vi "User Console.vi"(8 "error in":errorcluster) -> (0 "error out":errorcluster)   [LabVIEW 2020]
doc: "User Console thread VI"
uses:
  Controls/Events_User.ctl
  Database/Controls/Account Database.ctl
  Controls/Data_Initialize.ctl
  SubVIs/User Event - Stop/User Event - Stop.lvlib
  <vilib>/Utility/error.llb/Error Cluster From Error Code.vi
  <vilib>/ErrorRing/Error Ring.xnode
  SubVIs/Message Queue/Message Queue.lvlib
  SubVIs/Message Queue/Enqueue Message (Single).vi
  FGV/Controls/FGV_State.ctl
  Controls/User Console references.ctl
  Controls/User console Local Data.ctl
  Controls/Keypad.ctl
  Controls/Transactions.ctl
  Controls/User Console.ctl
panel:
  in  "User Console":T1
  # "[Covers: UI2]"
  # "[Covers: UI1]"
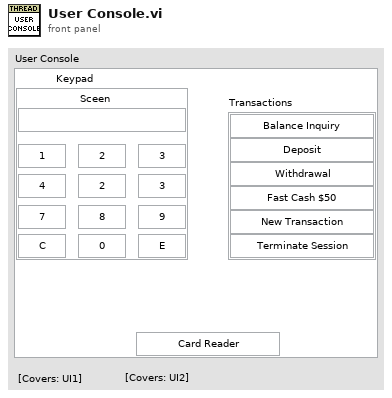
[diagram p1: front panel]
types:
  T1 = typedef "User Console.ctl" = cluster{"Keypad":T2, "Transactions":T3, "Card Reader":bool}
  T2 = typedef "Keypad.ctl" = cluster{"Sceen":string, "1":bool, "2":bool, "3":bool, "4":bool, "5":bool, "6":bool, "7":bool, "8":bool, "9":bool, "C":bool, "0":bool, "E":bool}
  T3 = typedef "Transactions.ctl" = cluster{"Balance Inquiry":bool, "Deposit":bool, "Withdrawal":bool, "Fast Cash $50":bool, "New Transaction":bool, "Terminate Session":bool}
  T4 = enum32{"Invalid", "Standard", "Closed", "Hidden", "Minimized", "Maximized"}
  T5 = typedef "FGV_State.ctl" = enum16{"1 - OpenDatabase", "2 - Initialize Events", "3 - Initialize QMH", "4 - Close QMH", "5 - Close Events", "Read FGV", "Save Database", "Def"}
  T6 = typedef "FGV_Data.ctl" = cluster{"QMH":T7, "User Events":T8, "Database":T9[]}
  T7 = typedef "Message Queue.lvlib/All Message Queues.ctl" = cluster{"User Console":refnum<queue>, "Display Console":refnum<queue>, "Sensor Interface":refnum<queue>, "Process":refnum<queue>}
  T8 = typedef "Events_User.ctl" = cluster{"Stop User Console":refnum<user-event>, "Error User Console":refnum<user-event>, "Stop Sensor Interface ":refnum<user-event>, "Error Sensor Interface":refnum<user-event>}
  T9 = typedef "Account Database.ctl" = cluster{"Account Number":i32, "First Name":string, "Last Name":string, "Balance":dbl}
  T10 = typedef "User console Local Data.ctl" = cluster{"Initiliaze":T11, "User Console Ref":T12, "Configuration Database":T9}
  T11 = typedef "Data_Initialize.ctl" = cluster{"Database":T9[], "User Events":T8}
  T12 = typedef "User Console references.ctl" = cluster{"0":refnum<vi>, "1":refnum<vi>, "2":refnum<vi>, "3":refnum<vi>, "4":refnum<vi>, "5":refnum<vi>, "6":refnum<vi>, "7":refnum<vi>, "8":refnum<vi>, "9":refnum<vi>, "Deposit":refnum<vi>, "Fast Cash $50":refnum<vi>, "Balance Inquiry":refnum<vi>, "Sceen":refnum<vi>, "Card Reader":refnum<vi>, "Withdrawal":refnum<vi>, "New Transaction":refnum<vi>, "Terminate Session":refnum<vi>, "E":refnum<vi>, "C":refnum<vi>}
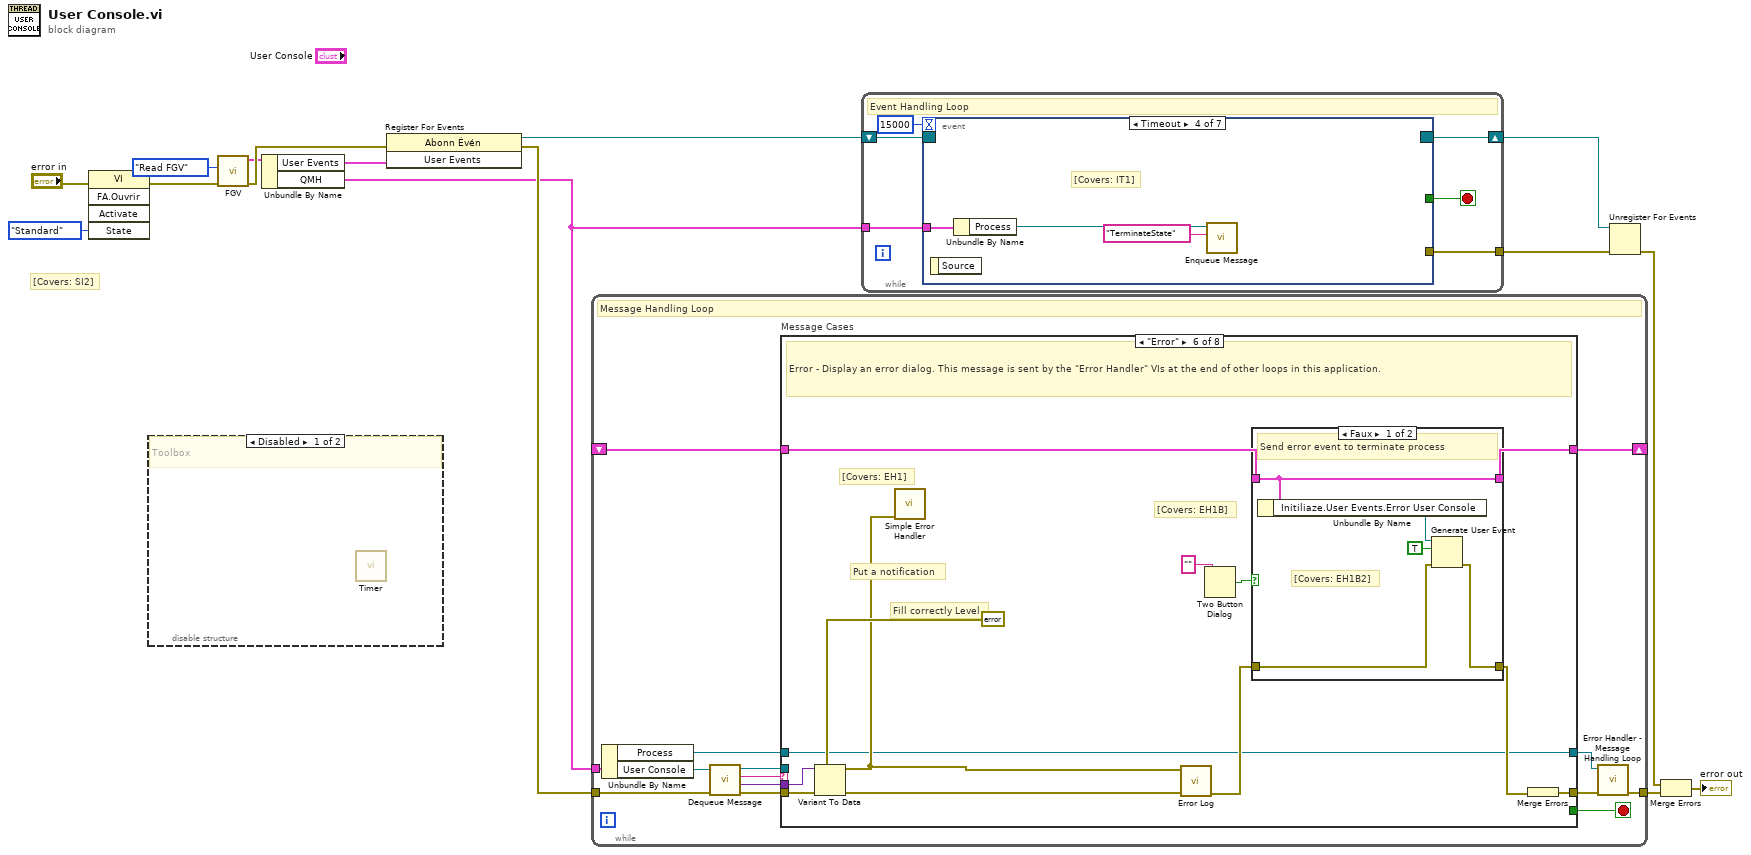
[diagram p0: block diagram]
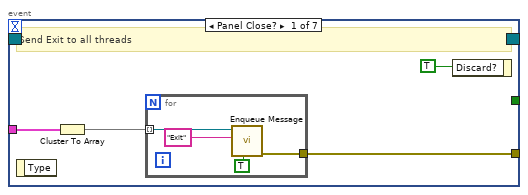
[diagram p3: hidden frame]
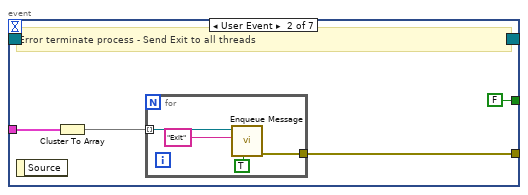
[diagram p4: hidden frame]
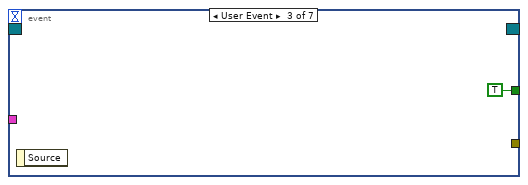
[diagram p5: hidden frame]
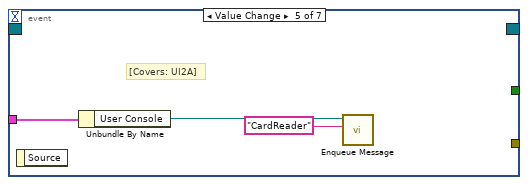
[diagram p6: hidden frame]
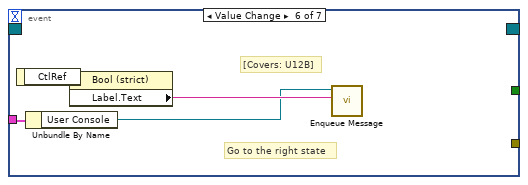
[diagram p7: hidden frame]
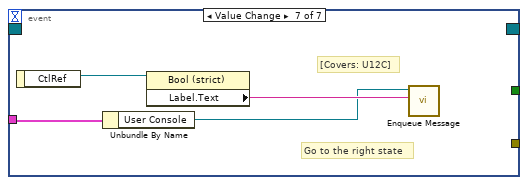
[diagram p8: hidden frame]
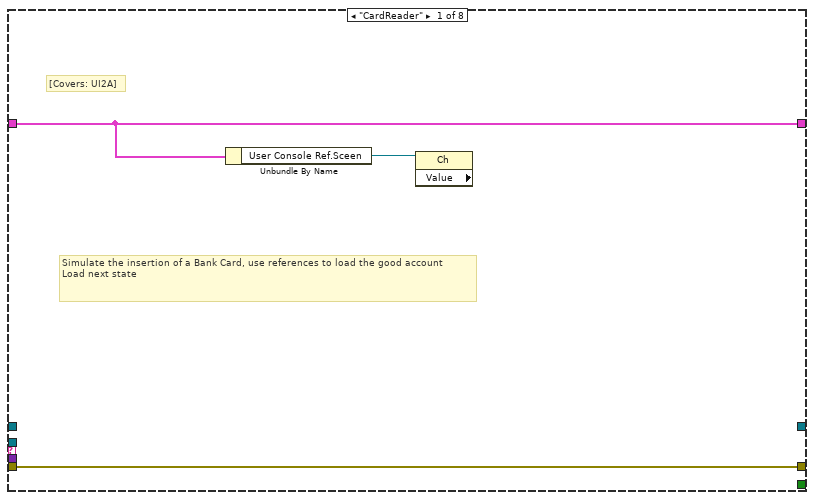
[diagram p9: hidden frame]
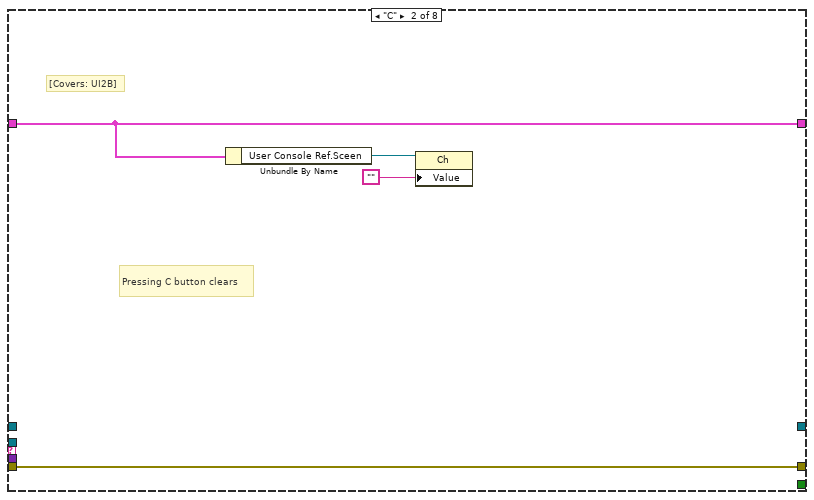
[diagram p10: hidden frame]
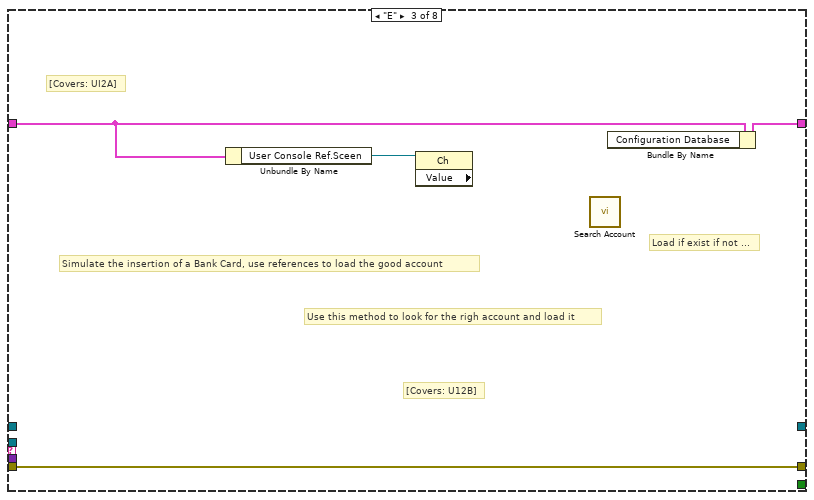
[diagram p11: hidden frame]
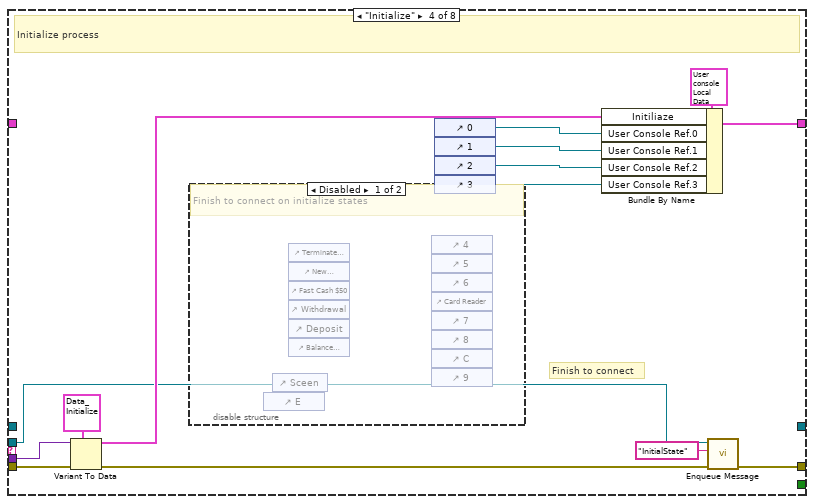
[diagram p12: hidden frame]
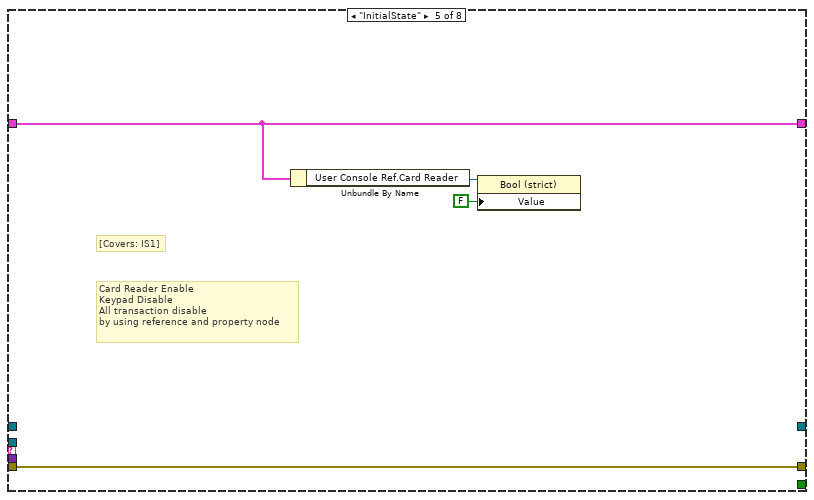
[diagram p14: hidden frame]
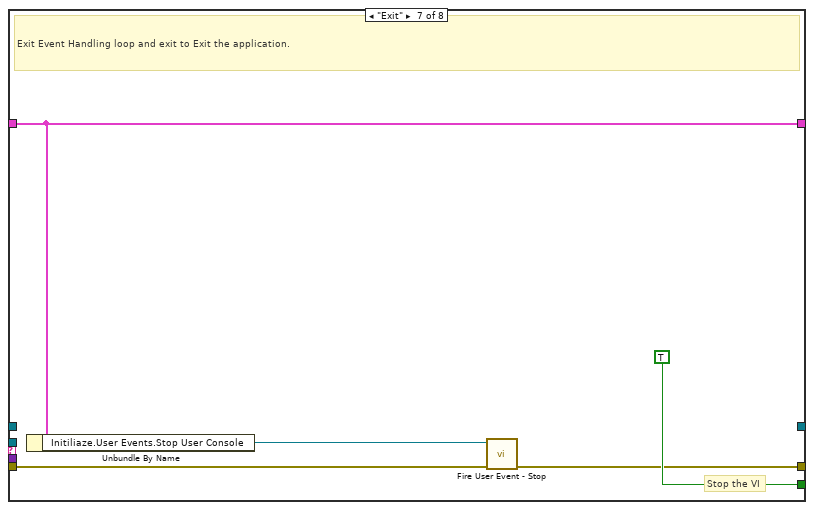
[diagram p16: hidden frame]
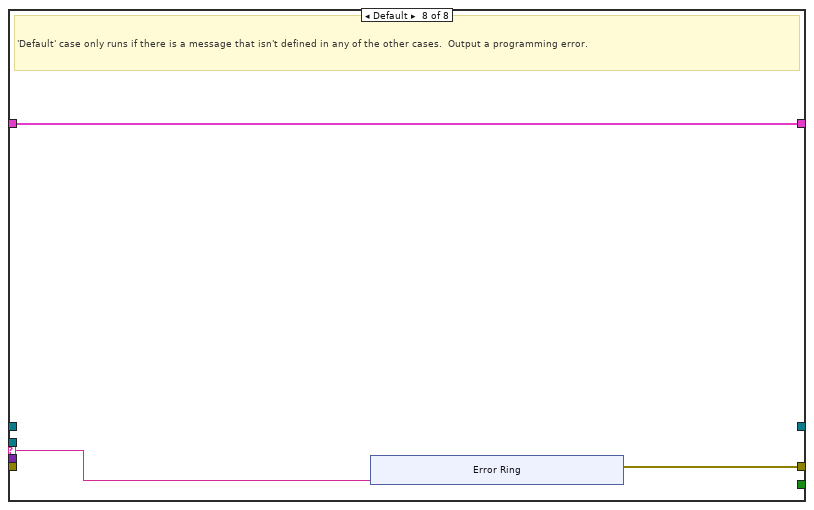
[diagram p17: hidden frame]
diagram:
  # "[Covers: SI2]"
  n1 = invoke class="VI" method="FA.Ouvrir"(error in="error in", "State"=T4."Standard") -> (error out=w2:errorcluster)  [unwired: 3 in, 4 out]
  n2 = disable-structure shown="Disabled" {
    frame Disabled {
      # "Toolbox"
      n3 = call "Timer.vi"() -> ()  [unwired: 9 in, 3 out]
    }
    frame Enabled {
    }
  }
  n4 = call "FGV.vi"("error in (no error)"=w2, "FGV_State"=FGV_State."Read FGV") -> ("error out"=w12:errorcluster, "FGV"=w10:T6)  [unwired: 8 in]
  n5 = Unbundle By Name(w10) -> ("User Events"=w11:T8, "QMH"=w14:T7)
  n6 = register-events(error in=w12, w11) -> (reference out=w8:refnum<event-registration>, error out=w15:errorcluster)  [unwired: 1 in]
  n7 = while {
    tunnel: w14 -> [w19]
    shift-right: [w28] -> _
    shift-left: _ -> [w29]
    tunnel: w15 -> [w26]
    tunnel: [w21] -> w4
    stop <- w27 stop-if-true
    # "Message Handling Loop"
    n8 = Unbundle By Name(w19) -> ("Process"=w17:refnum<queue>, "User Console"=w18:refnum<queue>)
    n9 = call "Dequeue Message.vi"("error in (no error)"=w26, "Message Queue"=w18) -> ("error out"=w25:errorcluster, "Message Data"=w23:variant, "Message"=w24:string, "dup Message Queue"=w22:refnum<queue>)  [unwired: 6 in]
    n10 = case "Message Cases" shown="\"Error\"" w24 {
      selector: w24 -> [_ _ _ _ _ _ _ w84]
      tunnel: w22 -> [_ _ _ w42 _ _ _ _]
      tunnel: w25 -> [w32 w36 w40 w53 w58 w71 w80 _]
      tunnel: [w32 w36 w40 w41 w58 w68 w79 w85] -> w20
      tunnel: w29 -> [w30 w34 w39 _ w57 w62 w82 w86]
      tunnel: [w30 w34 w37 w54 w57 w61 w82 w86] -> w28
      tunnel: [_ _ _ _ _ _ TRUE _] -> w27
      tunnel: w23 -> [_ _ _ w50 _ w70 _ _]
      tunnel: w17 -> [_ _ _ _ _ w59 _ _]
      tunnel: [_ _ _ _ _ w59 _ _] -> w16
      frame "CardReader" {
        # "Simulate the insertion of a Bank Card, use references to load the good account\nLoad next state"
        # "[Covers: UI2A]"
        n11 = Unbundle By Name(w30) -> ("User Console Ref.Sceen"=w31:refnum<vi>)
        n12 = property class="Ch" props=["Value"](reference=w31) -> ()  [unwired: 1 in, 3 out]
      }
      frame "C" {
        # "Pressing C button clears"
        # "[Covers: UI2B]"
        n13 = Unbundle By Name(w34) -> ("User Console Ref.Sceen"=w35:refnum<vi>)
        n14 = property class="Ch"(reference=w35, "Value"="") -> ()  [unwired: 1 in, 2 out]
      }
      frame "E" {
        # "[Covers: U12B]"
        # "Load if exist if not ..."
        # "Use this method to look for the righ account and load it"
        # "Simulate the insertion of a Bank Card, use references to load the good account"
        # "[Covers: UI2A]"
        n15 = Unbundle By Name(w39) -> ("User Console Ref.Sceen"=w38:refnum<vi>)
        n16 = property class="Ch" props=["Value"](reference=w38) -> ()  [unwired: 1 in, 3 out]
        n17 = call "Search Account.vi"() -> ()  [unwired: 9 in, 3 out]
        n18 = Bundle By Name(cluster=w39) -> (w37:T10)  [unwired: 1 in]
      }
      frame "Initialize" {
        # "Finish to connect"
        # "Initialize process"
        n19 = Variant To Data(error in=w53, type=T11 {"Database"=[], "User Events"={"Stop User Console"=refnum, "Error User Console"=refnum, "Stop Sensor Interface "=refnum, "Error Sensor Interface"=refnum}} ("Initiliaze"), Variant=w50) -> (data=w51:T11, error out=w43:errorcluster)
        n20 = disable-structure shown="Disabled" {
          frame Disabled {
            # "Finish to connect on initialize states"
            n21 = control-ref of="E"() -> ()  [unwired: 1 out]
            n22 = control-ref of="Sceen"() -> ()  [unwired: 1 out]
            n23 = control-ref of="Terminate Session"() -> ()  [unwired: 1 out]
            n24 = control-ref of="New Transaction"() -> ()  [unwired: 1 out]
            n25 = control-ref of="Fast Cash $50"() -> ()  [unwired: 1 out]
            n26 = control-ref of="Withdrawal"() -> ()  [unwired: 1 out]
            n27 = control-ref of="Deposit"() -> ()  [unwired: 1 out]
            n28 = control-ref of="Balance Inquiry"() -> ()  [unwired: 1 out]
            n29 = control-ref of="4"() -> ()  [unwired: 1 out]
            n30 = control-ref of="5"() -> ()  [unwired: 1 out]
            n31 = control-ref of="6"() -> ()  [unwired: 1 out]
            n32 = control-ref of="Card Reader"() -> ()  [unwired: 1 out]
            n33 = control-ref of="7"() -> ()  [unwired: 1 out]
            n34 = control-ref of="8"() -> ()  [unwired: 1 out]
            n35 = control-ref of="C"() -> ()  [unwired: 1 out]
            n36 = control-ref of="9"() -> ()  [unwired: 1 out]
          }
          frame Enabled {
          }
        }
        n37 = control-ref of="0"() -> (w48:refnum<vi>)
        n38 = control-ref of="1"() -> (w47:refnum<vi>)
        n39 = control-ref of="2"() -> (w46:refnum<vi>)
        n40 = control-ref of="3"() -> (w45:refnum<vi>)
        n41 = Bundle By Name(cluster=T10 {"Initiliaze"={"Database"=[], "User Events"={"Stop User Console"=refnum, "Error User Console"=refnum, "Stop Sensor Interface "=refnum, "Error Sensor Interface"=refnum}}, "User Console Ref"={"0"=refnum, "1"=refnum, "2"=refnum, "3"=refnum, "4"=refnum, "5"=refnum, "6"=refnum, "7"=refnum, "8"=refnum, "9"=refnum, "Deposit"=refnum, "Fast Cash $50"=refnum, "Balance Inquiry"=refnum, "Sceen"=refnum, "Card Reader"=refnum, "Withdrawal"=refnum, "New Transaction"=refnum, "Terminate Session"=refnum, "E"=refnum, "C"=refnum}, "Configuration Database"={"Account Number"=0, "First Name"="", "Last Name"="", "Balance"=0.0}} ("Local Data"), "Initiliaze"=w51, "User Console Ref.0"=w48, "User Console Ref.1"=w47, "User Console Ref.2"=w46, "User Console Ref.3"=w45) -> (w54:T10)
        n42 = call-poly "Enqueue Message.vi"("error in (no error)"=w43, "Message"="InitialState", "Message Queue"=w42) -> ("error out"=w41:errorcluster)  [unwired: 7 in, 1 out]
      }
      frame "InitialState" {
        # "Card Reader Enable\nKeypad Disable\nAll transaction disable\nby using reference and property node"
        # "[Covers: IS1]"
        n43 = Unbundle By Name(w57) -> ("User Console Ref.Card Reader"=w56:refnum<vi>)
        n44 = property class="Bool (strict)"(reference=w56, "Value"=FALSE) -> ()  [unwired: 1 in, 2 out]
      }
      frame "Error" {
        # "Put a notification"
        # "[Covers: EH1B]"
        # "[Covers: EH1]"
        # "Fill correctly Level"
        # "Error - Display an error dialog. This message is sent by the \"Error Handler\" VIs at the end of other loops in this application."
        n45 = Variant To Data(error in=w71, type=errorcluster {"status"=FALSE, "code"=0, "source"=""} ("error constant"), Variant=w70) -> (data=w66:errorcluster, error out=w67:errorcluster)
        n46 = call <vilib>:"Simple Error Handler.vi"("error in (no error)"=w66) -> ()  [unwired: 4 in, 5 out]
        n47 = call "Error Log.vi"("error in"=w67, "error happened"=w66) -> ("error out"=w65:errorcluster)  [unwired: 9 in]
        n48 = Two Button Dialog(message="") -> (T button?=w64:bool)  [unwired: 2 in]
        n49 = case shown="Faux" w64 {
          tunnel: w65 -> [w74 w78]
          tunnel: [w73 w78] -> w63
          tunnel: w62 -> [w76 w77]
          tunnel: [w76 w77] -> w61
          frame False {
            # "[Covers: EH1B2]"
            # "Send error event to terminate process"
            n50 = Unbundle By Name(w76) -> ("Initiliaze.User Events.Error User Console"=w75:refnum<user-event>)
            n51 = Generate User Event(user event=w75, event data cluster=TRUE ("event data"), error in=w74) -> (error out=w73:errorcluster)  [unwired: 1 in, 1 out]
          }
          frame True {
            # "[Covers: EH1B1]"
            # "Continu (ok)"
          }
        }
        n52 = Merge Errors(w63) -> (w68:errorcluster)
      }
      frame "Exit" {
        # "Stop the VI"
        # "Exit Event Handling loop and exit to Exit the application."
        n53 = Unbundle By Name(w82) -> ("Initiliaze.User Events.Stop User Console"=w81:refnum<user-event>)
        n54 = call "Fire User Event - Stop.vi"("error in (no error)"=w80, "User Event - Stop"=w81) -> ("error out"=w79:errorcluster)  [unwired: 9 in]
      }
      frame Default {
        # "'Default' case only runs if there is a message that isn't defined in any of the other cases.  Output a programming error."
        n55 = xnode "Error Ring"("paramètre 0"=w84) -> ("sortie d'erreur"=w85:errorcluster)
      }
    }
    n56 = call "Error Handler - Message Handling Loop.vi"("error in (no error)"=w20, "Message Queue"=w16) -> ("dup error in"=w21:errorcluster)  [unwired: 8 in, 1 out]
  }
  n57 = while {
    tunnel: w14 -> [w99]
    shift-right: [w97] -> w6
    shift-left: w8 -> [w98]
    tunnel: [w95] -> w7
    stop <- w96 stop-if-true
    # "Event Handling Loop"
    n58 = event shown="[3] Timeout" {
      selector: w98 -> [_ _ _ _ _ _ _]
      dyn-events: [_ _ _ _ _ _ _] -> w97
      timeout: 15000 -> [_ _ _ _ _ _ _]
      tunnel: [_ FALSE ("Discard?") TRUE ("Discard?") _ _ _ _] -> w96
      tunnel: w99 -> [w102 w111 _ w118 w120 w124 w127]
      tunnel: [w101 w110 _ _ _ _ _] -> w95
      event Panel Close? {
        # "Send Exit to all threads"
        n59 = event-data() -> ()  [unwired: 1 in, 1 out]
        n60 = Cluster To Array(cluster=w102) -> (array=w100:refnum<queue>[])
        n61 = for {
          tunnel: w100 -> [w107] mode=indexing
          tunnel: [w106] -> w101
          n62 = call-poly "Enqueue Message.vi"("Priority Message? (F)"=TRUE, "Message"="Exit", "Message Queue"=w107) -> ("error out"=w106:errorcluster)  [unwired: 7 in, 1 out]
        }
        n63 = event-data("Discard?"=TRUE) -> ()  [unwired: 1 in, 1 out]
      }
      event User Event {
        # "Error terminate process - Send Exit to all threads"
        n64 = event-data() -> ()  [unwired: 1 in, 1 out]
        n65 = Cluster To Array(cluster=w111) -> (array=w109:refnum<queue>[])
        n66 = for {
          tunnel: w109 -> [w115] mode=indexing
          tunnel: [w114] -> w110
          n67 = call-poly "Enqueue Message.vi"("Priority Message? (F)"=TRUE, "Message"="Exit", "Message Queue"=w115) -> ("error out"=w114:errorcluster)  [unwired: 7 in, 1 out]
        }
      }
      event User Event {
        n68 = event-data() -> ()  [unwired: 1 in, 1 out]
      }
      event Timeout {
        # "[Covers: IT1]"
        n69 = event-data() -> ()  [unwired: 1 in, 1 out]
        n70 = Unbundle By Name(w118) -> ("Process"=w117:refnum<queue>)
        n71 = call-poly "Enqueue Message.vi"("Message"="TerminateState", "Message Queue"=w117) -> ()  [unwired: 8 in, 2 out]
      }
      event Value Change {
        # "[Covers: UI2A]"
        n72 = event-data() -> ()  [unwired: 1 in, 1 out]
        n73 = Unbundle By Name(w120) -> ("User Console"=w121:refnum<queue>)
        n74 = call-poly "Enqueue Message.vi"("Message"="CardReader", "Message Queue"=w121) -> ()  [unwired: 8 in, 2 out]
      }
      event Value Change {
        # "[Covers: U12B]"
        # "Go to the right state"
        n75 = event-data() -> ("CtlRef"=w126:refnum<vi>)  [unwired: 1 in]
        n76 = Unbundle By Name(w124) -> ("User Console"=w123:refnum<queue>)
        n77 = property class="Bool (strict)"(reference=w126) -> ("Label.Text"=w125:string)  [unwired: 1 in, 2 out]
        n78 = call-poly "Enqueue Message.vi"("Message"=w125, "Message Queue"=w123) -> ()  [unwired: 8 in, 2 out]
      }
      event Value Change {
        # "[Covers: U12C]"
        # "Go to the right state"
        n79 = event-data() -> ("CtlRef"=w128:refnum<vi>)  [unwired: 1 in]
        n80 = Unbundle By Name(w127) -> ("User Console"=w129:refnum<queue>)
        n81 = property class="Bool (strict)"(reference=w128) -> ("Label.Text"=w130:string)  [unwired: 1 in, 2 out]
        n82 = call-poly "Enqueue Message.vi"("Message"=w130, "Message Queue"=w129) -> ()  [unwired: 8 in, 2 out]
      }
    }
  }
  n83 = Unregister For Events(event registration refnum=w6, error in=w7) -> (error out=w5:errorcluster)
  n84 = Merge Errors(w5, w4) -> (→"error out":errorcluster)
